vi "Set Variant Label.vi"(6 "Use  default values? [F, copy values]":bool, 7 "Label":string, 8 "error in (no error)":errorcluster, 10 "Variant":variant, 11 "Carya Config in":refnum<class "Carya Config.lvclass">) -> (0 "error out":errorcluster, 2 "Variant":variant, 3 "Carya Config out":refnum<class "Carya Config.lvclass">)   [LabVIEW 2013, in "Carya Config.lvclass"]
doc: "Copyright 2018, Carya Automatisering, Wiebe Walstra."
uses:
  Carya Config.lvclass
  <vilib>/Utility/VariantDataType/VariantType.lvlib
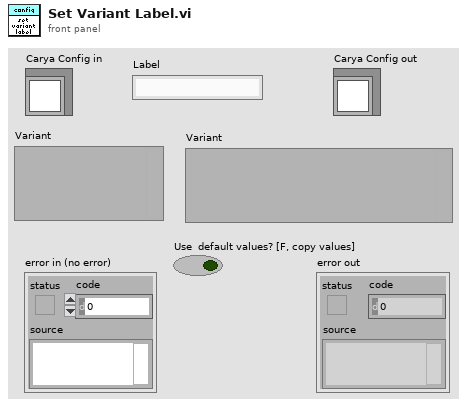
[diagram p1: front panel]
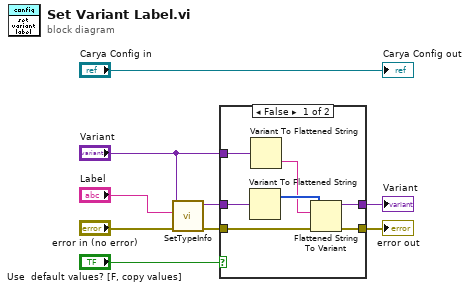
[diagram p0: block diagram]
diagram:
  n1 = call <vilib>:"SetTypeInfo.vi"("error in (no error)"="error in (no error)", "Name"="Label", "Variant"="Variant") -> ("error out"=w5:errorcluster, "Variant Out"=w3:variant)  [unwired: 7 in]
  n2 = case shown="False" "Use  default values? [F, copy values]" {
    tunnel: "Variant" -> [w16 _]
    tunnel: w5 -> [w15 w18]
    tunnel: [w14 w18] -> w4
    tunnel: w3 -> [w13 w17]
    tunnel: [w10 w17] -> w2
    frame False {
      n3 = Variant To Flattened String(Variant=w13) -> (1:w12:i16[])  [unwired: 1 out]
      n4 = Variant To Flattened String(Variant=w16) -> (data string=w11:string)  [unwired: 1 out]
      n5 = Flattened String To Variant(4:w15, 6:w11, 7:w12) -> (0:w14:errorcluster, 3:w10:variant)
    }
    frame True {
    }
  }
  "error out" <- w4
  "Variant" <- w2
  "Carya Config out" <- "Carya Config in"
